vi "multiPlots.vi"() -> ()   [LabVIEW 2016]
panel:
  in  "y axis":u16(ring)=3 items=["time", "rate of change of B", "magnetic field", "signal A", "signal B", "1/B"]
  in  "x axis":u16(ring)=2 items=["time", "rate of change of B", "magnetic field", "signal A", "signal B", "1/B"]
  in  "?":bool
  out "plotted data":cluster{dbl[], dbl[]}[](graph)
  # "rising"
  # "falling"
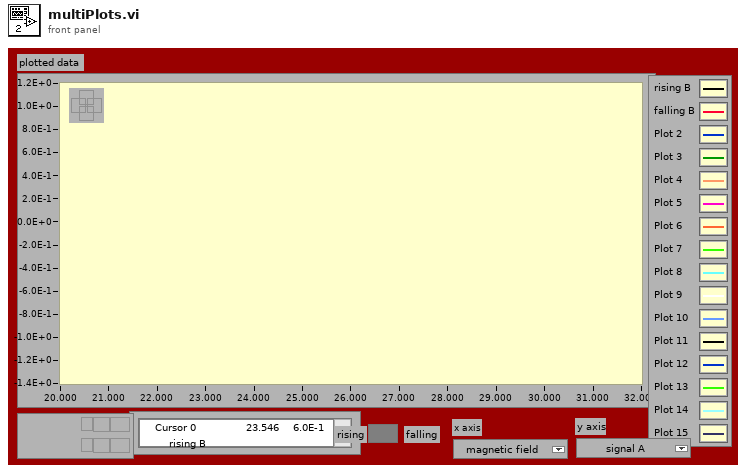
[diagram p1: front panel]
types:
  T1 = cluster{"ch B falling":dbl[], "ch B falling":dbl[]}
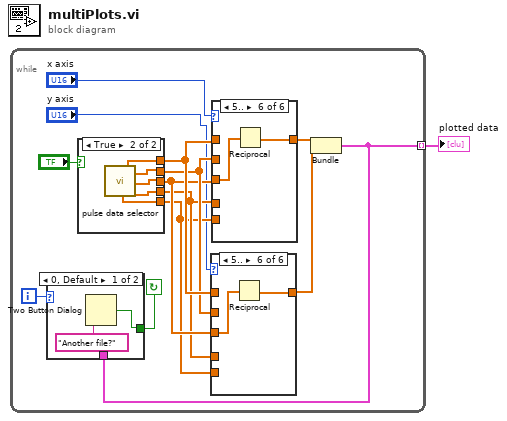
[diagram p0: block diagram]
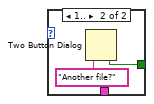
[diagram p2: hidden frame]
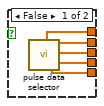
[diagram p13: hidden frame]
diagram:
  n1 = while {
    tunnel: [w2] -> w1 mode=indexing
    i -> [w4]
    stop <- w3 continue-if-true
    n2 = case shown="True" "?" {
      tunnel: [w37 w42] -> w13
      tunnel: [w36 w41] -> w12
      tunnel: [w35 w40] -> w11
      tunnel: [w34 w39] -> w10
      tunnel: [w33 w38] -> w9
      frame False {
        n3 = call "pulse data selector.vi"() -> ("time rising"=w37:dbl[], "ch B rising"=w33:dbl[], "dB/dt rising"=w36:dbl[], "B rising"=w35:dbl[], "ch A rising"=w34:dbl[])  [unwired: 7 in, 8 out]
      }
      frame True {
        n4 = call "pulse data selector.vi"() -> ("ch B falling"=w38:dbl[], "time falling"=w42:dbl[], "dB/dt falling"=w41:dbl[], "B falling"=w40:dbl[], "ch A falling"=w39:dbl[])  [unwired: 7 in, 8 out]
      }
    }
    n5 = case shown="5.." "y axis" {
      tunnel: w12 -> [_ w20 _ _ _ _]
      tunnel: w11 -> [_ _ w21 _ _ w24]
      tunnel: w10 -> [_ _ _ w22 _ _]
      tunnel: [w19 w20 w21 w22 w23 w25] -> w5
      tunnel: w9 -> [_ _ _ _ w23 _]
      tunnel: w13 -> [w19 _ _ _ _ _]
      frame ..0 {
      }
      frame 1 {
      }
      frame 2 {
      }
      frame 3 {
      }
      frame 4 {
      }
      frame 5.. {
        n6 = Reciprocal(x=w24) -> (1/x=w25:dbl[])
      }
    }
    n7 = case shown="5.." "x axis" {
      tunnel: w13 -> [w26 _ _ _ _ _]
      tunnel: w12 -> [_ w27 _ _ _ _]
      tunnel: w11 -> [_ _ w28 _ _ w31]
      tunnel: w10 -> [_ _ _ w29 _ _]
      tunnel: [w26 w27 w28 w29 w30 w32] -> w6
      tunnel: w9 -> [_ _ _ _ w30 _]
      frame ..0 {
      }
      frame 1 {
      }
      frame 2 {
      }
      frame 3 {
      }
      frame 4 {
      }
      frame 5.. {
        n8 = Reciprocal(x=w31) -> (1/x=w32:dbl[])
      }
    }
    n9 = Bundle("ch B falling"=w6, "ch B falling"=w5) -> (w2:T1)  [unwired: 1 in]
    n10 = case shown="0, Default" w4 {
      tunnel: [w15 w17] -> w3
      tunnel: w2 -> [_ _]
      frame 0, Default {
        n11 = Two Button Dialog(message="Another file?") -> (T button?=w15:bool)  [unwired: 2 in]
      }
      frame 1.. {
        n12 = Two Button Dialog(message="Another file?") -> (T button?=w17:bool)  [unwired: 2 in]
      }
    }
  }
  "plotted data" <- w1
